vi "GetTimeArrayAsDouble.vi"(9 "Get every n-th":i32, 11 "Waveform":waveform(dbl)) -> (3 "Time Array":dbl[](array[numeric]))   [LabVIEW 2019]
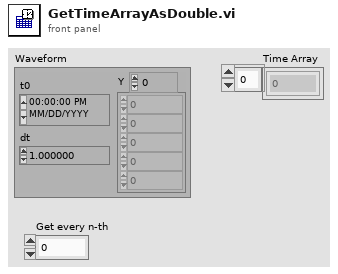
[diagram p1: front panel]
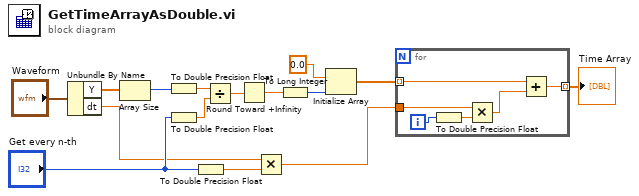
[diagram p0: block diagram]
diagram:
  n1 = Unbundle By Name("Waveform") -> ("Y"=w12:dbl[], "dt"=w2:dbl)
  n2 = Array Size(array=w12) -> (size(s)=w6:i32)
  n3 = To Double Precision Float(number=w6) -> (double precision float=w7:dbl)
  n4 = To Double Precision Float(number="Get every n-th") -> (double precision float=w8:dbl)
  n5 = To Double Precision Float(number="Get every n-th") -> (double precision float=w3:dbl)
  n6 = Divide(x=w7, y=w8) -> (x/y=w10:dbl)
  n7 = Round Toward +Infinity(x=w10) -> (ceil(x): smallest int >= x=w9:dbl)
  n8 = Multiply(x=w2, y=w3) -> (x*y=w1:dbl)
  n9 = To Long Integer(number=w9) -> (32bit integer=w5:i32)
  n10 = Initialize Array(0.0, w5) -> (w14:dbl[])
  n11 = for {
    tunnel: w14 -> [w17] mode=indexing
    tunnel: w1 -> [w20]
    tunnel: [w16] -> w15 mode=indexing
    i -> [w21]
    n12 = To Double Precision Float(number=w21) -> (double precision float=w19:dbl)
    n13 = Multiply(x=w20, y=w19) -> (x*y=w18:dbl)
    n14 = Add(x=w17, y=w18) -> (x+y=w16:dbl)
  }
  "Time Array" <- w15
